vi "2021-07-09.vi"() -> ()   [LabVIEW 2019]
panel:
  out "time":cluster{i32[], i32[]}[](graph)
  out "throughput":cluster{i32[], dbl[]}[](graph)
  out "message rate":cluster{i32[], dbl[]}[](graph)
  # "STM"
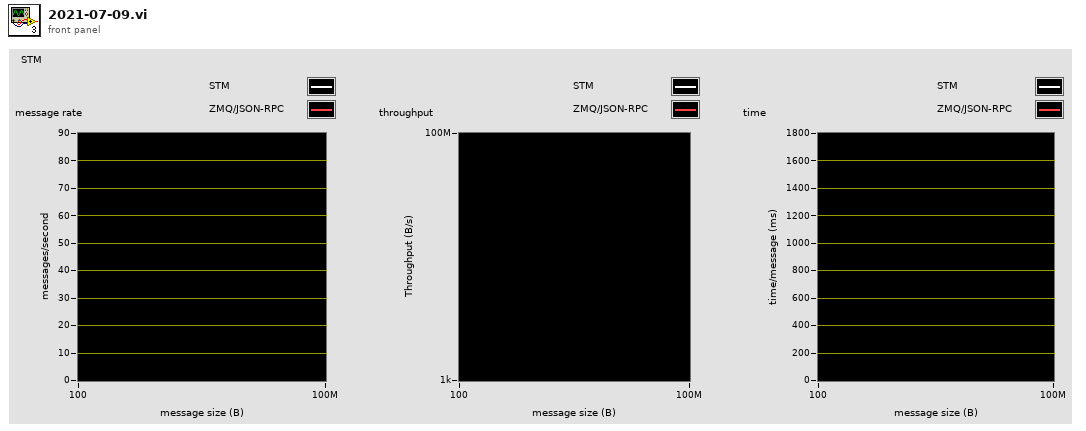
[diagram p1: front panel]
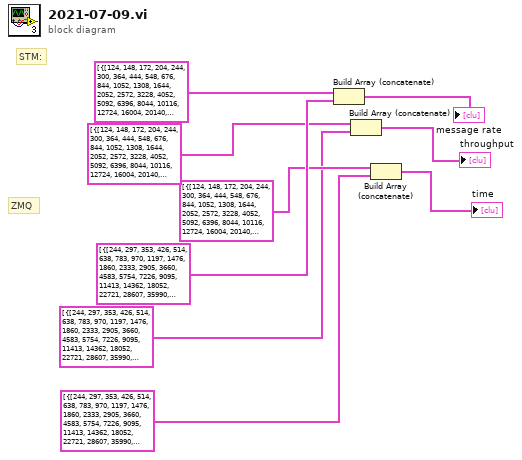
[diagram p0: block diagram]
diagram:
  # "ZMQ"
  # "STM:"
  n1 = Build Array (concatenate)(cluster{i32[], dbl[]}[] [{[124, 148, 172, 204, 244, 300, 364, 444, 548, 676, 844, 1052, 1308, 1644, 2052, 2572, 3228, 4052, 5092, 6396, 8044, 10116, 12724, 16004, 20140, 25340, 31892, 40140, 50524, 63588, 80044, 100756, 126836, 159668, 200996, 253028, 318532, 400996, 504812, 635508, 800044, 1007188, 1267956, 1596252, 2009556, 2529868, 3184900, 4009540, 5047700, 6354668, 8000044], [73.26007326007326, 37.31343283582089, 80.32128514056225, 80.97165991902834, 83.68200836820084, 81.30081300813008, 81.30081300813008, 81.30081300813008, 80.0, 81.9672131147541, 82.3045267489712, 82.98755186721992, 81.30081300813008, 82.98755186721992, 82.3045267489712, 80.64516129032258, 80.97165991902834, 81.9672131147541, 82.64462809917356, 82.64462809917356, 81.63265306122449, 80.0, 81.9672131147541, 82.64462809917356, 78.43137254901961, 82.3045267489712, 81.30081300813008, 80.64516129032258, 80.0, 80.0, 79.6812749003984, 79.6812749003984, 79.6812749003984, 75.18796992481202, 77.22007722007721, 74.07407407407408, 71.94244604316546, 69.68641114982579, 66.22516556291392, 62.30529595015576, 57.636887608069166, 50.125313283208015, 36.03603603603603, 31.84713375796178, 27.06359945872801, 23.80952380952381, 18.099547511312217, 13.89854065323141, 9.47867298578199, 7.163323782234958, 5.396654074473826]}] ("message rate"), cluster{i32[], dbl[]}[] [{[244, 297, 353, 426, 514, 638, 783, 970, 1197, 1476, 1860, 2333, 2905, 3660, 4583, 5754, 7226, 9095, 11413, 14362, 18052, 22721, 28607, 35990, 45262, 57027, 71748, 90267, 113711, 142986, 180100, 226656, 285362, 359078, 452157, 569307, 716716, 902172, 1135653, 1430011, 1799736, 2265809, 2852633, 3591256, 4521510, 5691835, 7165085, 9020945, 11356828, 14298020, 17999563], [60.42296072507553, 60.6060606060606, 60.6060606060606, 62.5, 63.09148264984227, 58.139534883720934, 65.359477124183, 68.4931506849315, 54.200542005420054, 62.11180124223603, 60.06006006006006, 65.78947368421053, 63.291139240506325, 51.41388174807198, 63.492063492063494, 64.1025641025641, 56.81818181818182, 65.14657980456026, 56.81818181818182, 54.94505494505495, 50.76142131979695, 49.26108374384236, 50.25125628140703, 49.75124378109452, 51.0204081632653, 44.54342984409799, 42.918454935622314, 40.48582995951417, 39.920159680638726, 37.38317757009346, 32.62642740619902, 28.40909090909091, 24.96878901373283, 21.141649048625794, 18.18181818181818, 14.388489208633095, 12.453300124533001, 10.655301012253597, 8.003201280512204, 6.736274840013473, 5.442176870748299, 4.519774011299435, 3.7064492216456637, 2.983738624496494, 2.384358607534573, 1.9719976336028398, 1.5360983102918588, 1.238927089140804, 0.963762528912876, 0.7363228039172374, 0.598623166716552]}] ("message rate 2")) -> (→"message rate":cluster{i32[], dbl[]}[])
  n2 = Build Array (concatenate)(cluster{i32[], dbl[]}[] [{[124, 148, 172, 204, 244, 300, 364, 444, 548, 676, 844, 1052, 1308, 1644, 2052, 2572, 3228, 4052, 5092, 6396, 8044, 10116, 12724, 16004, 20140, 25340, 31892, 40140, 50524, 63588, 80044, 100756, 126836, 159668, 200996, 253028, 318532, 400996, 504812, 635508, 800044, 1007188, 1267956, 1596252, 2009556, 2529868, 3184900, 4009540, 5047700, 6354668, 8000044], [9084.249084249084, 5522.388059701492, 13815.261044176706, 16518.218623481782, 20418.410041841005, 24390.243902439026, 29593.49593495935, 36097.560975609755, 43840.0, 55409.83606557377, 69465.02057613169, 87302.90456431535, 106341.46341463414, 136431.53526970954, 168888.8888888889, 207419.35483870967, 261376.51821862347, 332131.1475409836, 420826.4462809918, 528595.0413223141, 656653.0612244898, 809280.0, 1042950.8196721312, 1322644.6280991735, 1579607.843137255, 2085596.70781893, 2592845.5284552844, 3237096.7741935486, 4041920.0, 5087040.0, 6378007.96812749, 8028366.533864542, 10106454.183266932, 12005112.781954886, 15520926.64092664, 18742814.814814813, 22915971.22302158, 27943972.125435542, 33431258.278145697, 39595514.018691584, 46112046.10951009, 50485614.03508772, 45692108.1081081, 50836050.95541401, 54385818.673883624, 60234952.38095238, 57645248.86877828, 55726754.69075747, 47845497.630331755, 45520544.412607454, 43173470.04856989]}] ("throughput"), cluster{i32[], dbl[]}[] [{[244, 297, 353, 426, 514, 638, 783, 970, 1197, 1476, 1860, 2333, 2905, 3660, 4583, 5754, 7226, 9095, 11413, 14362, 18052, 22721, 28607, 35990, 45262, 57027, 71748, 90267, 113711, 142986, 180100, 226656, 285362, 359078, 452157, 569307, 716716, 902172, 1135653, 1430011, 1799736, 2265809, 2852633, 3591256, 4521510, 5691835, 7165085, 9020945, 11356828, 14298020, 17999563], [14743.202416918428, 18000.0, 21393.939393939392, 26625.0, 32429.022082018928, 37093.023255813954, 51176.470588235294, 66438.35616438357, 64878.04878048781, 91677.01863354037, 111711.7117117117, 153486.84210526317, 183860.7594936709, 188174.80719794345, 290984.126984127, 368846.1538461539, 410568.1818181818, 592508.1433224756, 648465.9090909092, 789120.8791208791, 916345.1776649746, 1119261.0837438423, 1437537.688442211, 1790547.263681592, 2309285.714285714, 2540178.1737193763, 3079313.30472103, 3654534.4129554657, 4539361.27744511, 5345271.028037383, 5876019.5758564435, 6439090.909090909, 7125143.570536829, 7591501.057082453, 8221036.363636363, 8191467.625899281, 8925479.452054795, 9612914.224826852, 9088859.543817526, 9632947.120242506, 9794481.632653061, 10240944.632768363, 10573139.362490734, 10715369.237654781, 10780901.287553648, 11224285.15085782, 11006274.961597543, 11176293.13014929, 10945285.27370856, 10527958.176864738, 10774955.402574081]}] ("throughput 2")) -> (→"throughput":cluster{i32[], dbl[]}[])
  n3 = Build Array (concatenate)(cluster{i32[], i32[]}[] [{[124, 148, 172, 204, 244, 300, 364, 444, 548, 676, 844, 1052, 1308, 1644, 2052, 2572, 3228, 4052, 5092, 6396, 8044, 10116, 12724, 16004, 20140, 25340, 31892, 40140, 50524, 63588, 80044, 100756, 126836, 159668, 200996, 253028, 318532, 400996, 504812, 635508, 800044, 1007188, 1267956, 1596252, 2009556, 2529868, 3184900, 4009540, 5047700, 6354668, 8000044], [14, 27, 12, 12, 12, 12, 12, 12, 12, 12, 12, 12, 12, 12, 12, 12, 12, 12, 12, 12, 12, 12, 12, 12, 13, 12, 12, 12, 12, 12, 13, 13, 13, 13, 13, 14, 14, 14, 15, 16, 17, 19, 27, 31, 36, 41, 54, 71, 104, 138, 183]}] ("time"), cluster{i32[], i32[]}[] [{[244, 297, 353, 426, 514, 638, 783, 970, 1197, 1476, 1860, 2333, 2905, 3660, 4583, 5754, 7226, 9095, 11413, 14362, 18052, 22721, 28607, 35990, 45262, 57027, 71748, 90267, 113711, 142986, 180100, 226656, 285362, 359078, 452157, 569307, 716716, 902172, 1135653, 1430011, 1799736, 2265809, 2852633, 3591256, 4521510, 5691835, 7165085, 9020945, 11356828, 14298020, 17999563], [17, 16, 16, 16, 16, 17, 15, 15, 18, 16, 17, 15, 16, 19, 16, 16, 18, 15, 18, 18, 20, 20, 20, 20, 20, 22, 23, 25, 25, 27, 31, 35, 40, 47, 55, 70, 80, 94, 125, 148, 183, 221, 269, 335, 418, 506, 650, 805, 1035, 1355, 1666]}] ("time 2")) -> (→"time":cluster{i32[], i32[]}[])
